vi "Initiate Session.vi"(8 "error in (no error)":errorcluster, 11 "SerialDriver in":refnum<class "SerialDriver.lvclass">) -> (0 "error out":errorcluster, 3 "SerialDriver out":refnum<class "SerialDriver.lvclass">)   [LabVIEW 2023, in "HAF.lvlib" / "SerialDriver.lvclass"]
doc: "Creates a Session for the Instrument that will be communicated with."
uses:
  SerialDriver.lvclass
  SerialDriver.lvclass/SerialDriver.ctl
  Driver/Driver.lvclass
  <vilib>/Instr/_visa.llb/VISA Configure Serial Port (Instr).vi
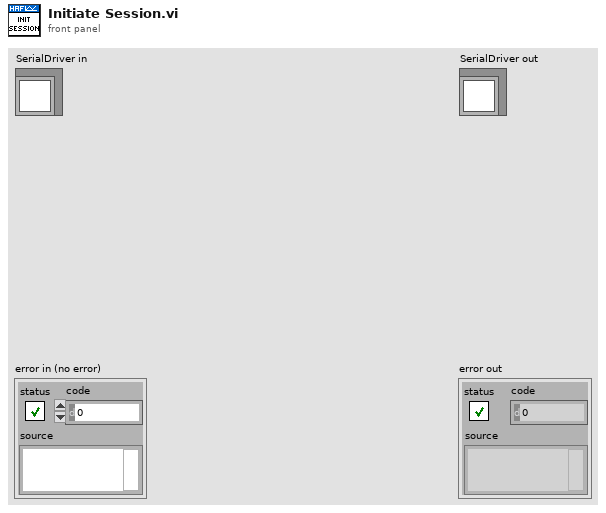
[diagram p1: front panel]
types:
  T1 = typedef "HAF.lvlib/Serial Port Attributes.ctl" = cluster{"Baud Rate":u32, "Data Bits":u16, "Stop Bits":u16, "Data Flow":u16, "Timeout":u32, "parity (0:none)":enum16{"None", "Odd", "Even", "Mark", "Space"}, "Establish Wait":u32}
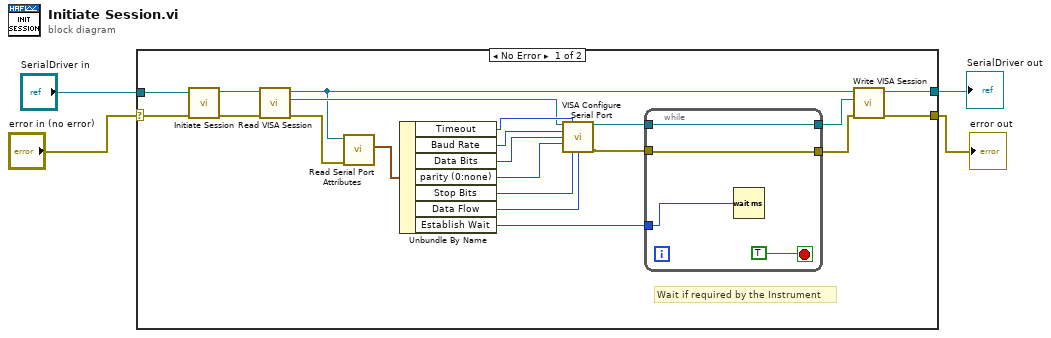
[diagram p0: block diagram]
diagram:
  n1 = case shown="No Error" "error in (no error)" {
    selector: "error in (no error)" -> [w24 w30]
    tunnel: "SerialDriver in" -> [w25 w31]
    tunnel: [w6 w31] -> w2
    tunnel: [w5 w30] -> w1
    frame No Error {
      # "Wait if required by the Instrument"
      n2 = call-parent "Initiate Session.vi"("error in (no error)"=w24, "Driver in"=w25) -> ("error out"=w22:errorcluster, "Driver out"=w23:refnum<class "SerialDriver.lvclass">)  [unwired: 8 in]
      n3 = call-dynamic "Read VISA Session.vi"("error in (no error)"=w22, "Driver in"=w23) -> ("error out"=w21:errorcluster, "VISA Session"=w10:refnum<visa-resource-name>, "Driver out"=w9:refnum<class "SerialDriver.lvclass">)  [unwired: 7 in]
      n4 = call-dynamic "Read Serial Port Attributes.vi"("error in (no error)"=w21, "SerialDriver in"=w9) -> ("Serial Port Attributes"=w20:T1)  [unwired: 7 in, 2 out]
      n5 = Unbundle By Name(w20) -> ("Timeout"=w15:u32, "Baud Rate"=w19:u32, "Data Bits"=w18:u16, "parity (0:none)"=w14:enum16{"None", "Odd", "Even", "Mark", "Space"}, "Stop Bits"=w17:u16, "Data Flow"=w16:u16, "Establish Wait"=w11:u32)
      n6 = call-poly "VISA Configure Serial Port"("VISA resource name"=w10, "timeout (10sec)"=w15, "baud rate (9600)"=w19, "data bits (8)"=w18, "parity (0:none)"=w14, "stop bits (10: 1 bit)"=w17, "flow control (0:none)"=w16) -> ("VISA resource name out"=w13:refnum<visa-resource-name>, "error out"=w12:errorcluster)  [unwired: 7 in]
      n7 = while {
        tunnel: w13 -> [w26]
        tunnel: w12 -> [w27]
        tunnel: w11 -> [w29]
        tunnel: [w27] -> w7
        tunnel: [w26] -> w8
        stop <- TRUE stop-if-true
        n8 = Wait (ms)(milliseconds to wait=w29) -> ()  [unwired: 1 out]
      }
      n9 = call-dynamic "Write VISA Session.vi"("error in (no error)"=w7, "VISA Session"=w8, "Driver in"=w9) -> ("error out"=w5:errorcluster, "Driver out"=w6:refnum<class "SerialDriver.lvclass">)  [unwired: 7 in]
    }
    frame Error {
    }
  }
  "error out" <- w1
  "SerialDriver out" <- w2
